vi "SimpleGit_Global_Interface.vi"() -> (3 "InterfaceTable":T1)   [LabVIEW 2017]
uses:
  <resource>/Framework/Providers/API/Global_Interface.ctl
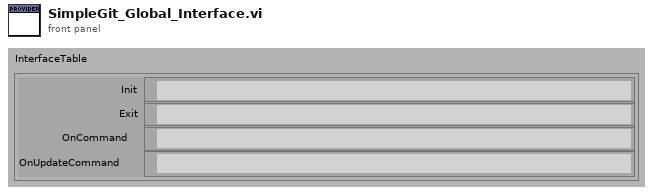
[diagram p1: front panel]
types:
  T1 = typedef "Global_Interface.ctl" = cluster{"Init":path, "Exit":path, "OnCommand":path, "OnUpdateCommand":path}
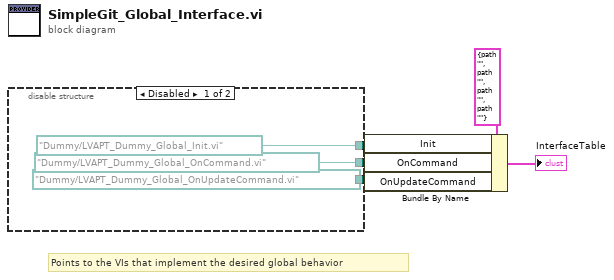
[diagram p0: block diagram]
diagram:
  # "Points to the VIs that implement the desired global behavior"
  n1 = disable-structure shown="Disabled" {
    disable-tunnel: [path "Dummy/LVAPT_Dummy_Global_OnCommand.vi" _] -> w3
    disable-tunnel: [path "Dummy/LVAPT_Dummy_Global_Init.vi" _] -> w2
    disable-tunnel: [path "Dummy/LVAPT_Dummy_Global_OnUpdateCommand.vi" _] -> w1
    frame Disabled {
    }
    frame Enabled {
    }
  }
  n2 = Bundle By Name(cluster=T1 {"Init"=path "", "Exit"=path "", "OnCommand"=path "", "OnUpdateCommand"=path ""} ("InterfaceTable"), "Init"=w2, "OnCommand"=w3, "OnUpdateCommand"=w1) -> (→"InterfaceTable":T1)
